vi "CS String to Num Array.vi"(11 "String":string) -> (1 "Positions":i32[](array[numeric]))   [LabVIEW 2024, in "Ocean Optics 2000 4000.lvlib"]
doc: "Scans a comma separated string into an array of numbers"
uses:
  Ocean Optics 2000 4000.lvlib
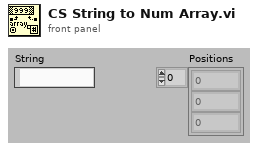
[diagram p1: front panel]
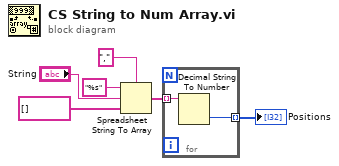
[diagram p0: block diagram]
diagram:
  n1 = Spreadsheet String To Array(delimiter (Tab)=",", format string="%s", spreadsheet string="String", array type (2D Dbl)=string[] []) -> (array=w4:string[])
  n2 = for {
    tunnel: [w8] -> w6 mode=indexing
    tunnel: w4 -> [w7] mode=indexing
    n3 = Decimal String To Number(string=w7) -> (number=w8:i32)  [unwired: 2 in, 1 out]
  }
  "Positions" <- w6
